vi "Ring to Text.vi"(1 "Ring ref":refnum<vi>) -> (0 "Text":string)   [LabVIEW 2015]
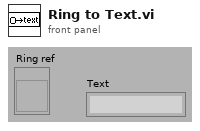
[diagram p1: front panel]
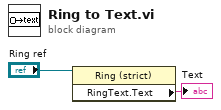
[diagram p0: block diagram]
diagram:
  n1 = property class="Ring (strict)"(reference="Ring ref") -> ("RingText.Text"=→"Text":string)  [unwired: 1 in, 2 out]
